vi "pyWebscraper.vi"(8 "error in":errorcluster, 11 "Functions":T1=enum."Check_Ratio") -> (0 "error out":errorcluster, 1 "2D Array":string[][](array[string]), 2 "Standard Output":string, 3 "Output":bool)   [LabVIEW 2025]
uses:
  Control/Function Enum.ctl
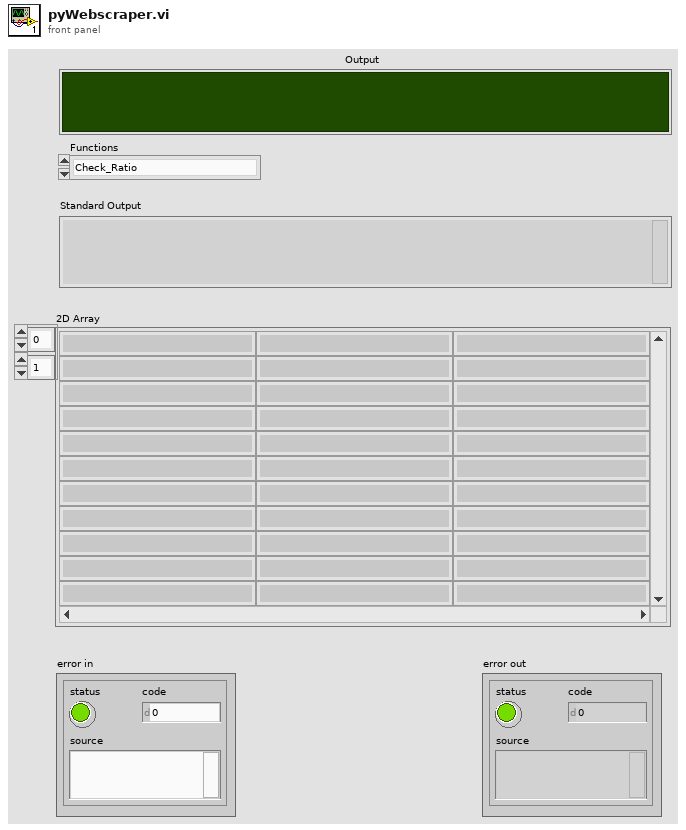
[diagram p1: front panel]
types:
  T1 = typedef "Function Enum.ctl" = enum16{"Check_Config", "Check_Security", "Check_Ratio", "Check_GUI_Loaded", "Read_Overview", "Read_Parameters", "Read_Events", "Read_Alarm", "Read_Settings", "Config_All_Port_Default", "Config_Port1_Speed_10M", "Config_Port1_Speed_100M", "Config_Port2_Speed_10M", "Config_Port2_Speed_100M"}
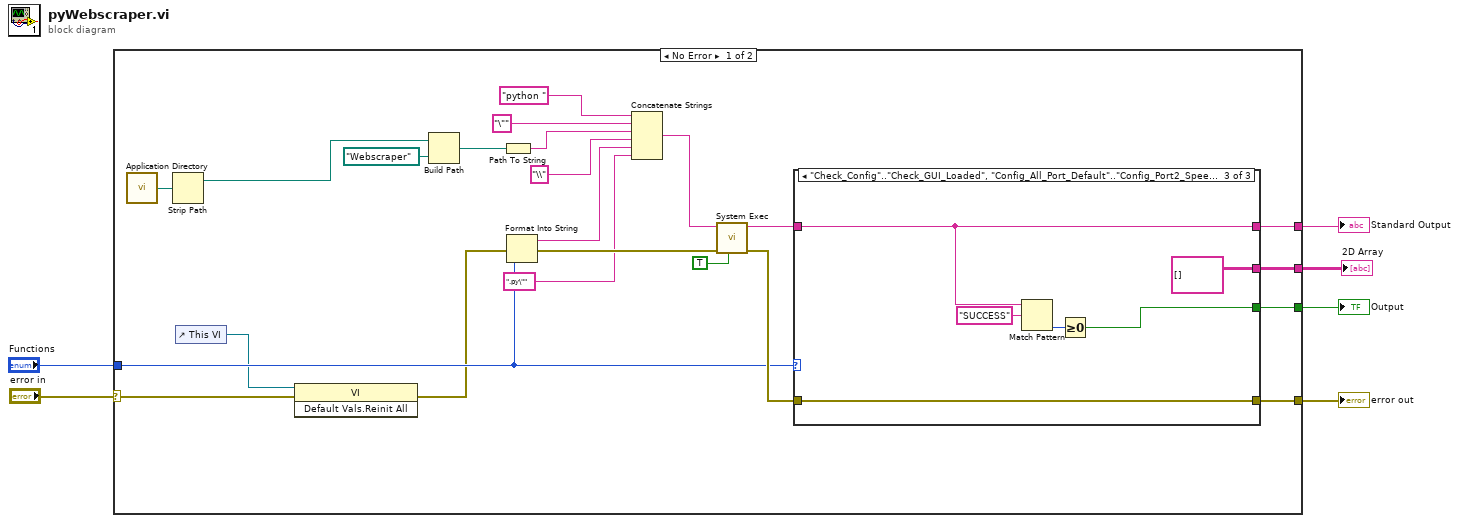
[diagram p0: block diagram]
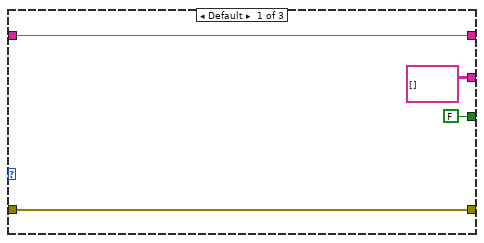
[diagram p2: hidden frame]
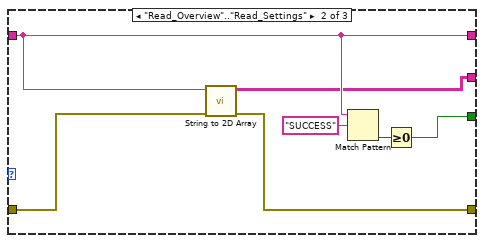
[diagram p3: hidden frame]
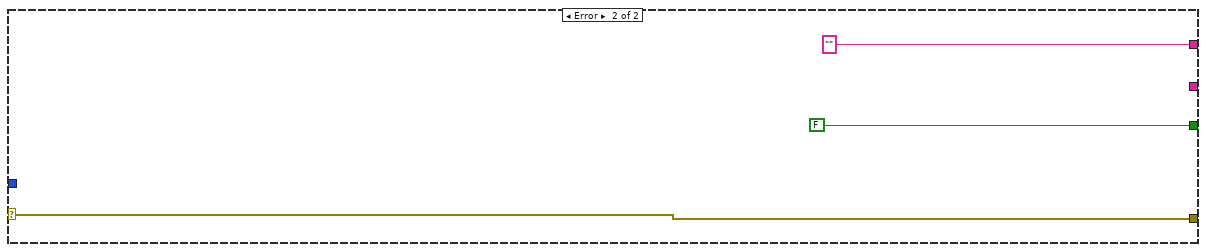
[diagram p4: hidden frame]
diagram:
  n1 = case shown="No Error" "error in" {
    selector: "error in" -> [w8 w49]
    tunnel: [w23 w49] -> w5
    tunnel: "Functions" -> [w22 _]
    tunnel: [w20 "" ("standard output")] -> w4
    tunnel: [w21 FALSE] -> w3
    tunnel: [w19 _] -> w1
    frame No Error {
      n2 = call <vilib>:"Application Directory.vi"() -> ("Application Directory"=w29:path)
      n3 = Strip Path(path=w29) -> (stripped path=w17:path)  [unwired: 1 out]
      n4 = control-ref of="This VI"() -> (w9:refnum<vi>)
      n5 = invoke class="VI" method="Default Vals.Reinit All"(reference=w9, error in=w8) -> (error out=w7:errorcluster)  [unwired: 1 in, 2 out]
      n6 = Build Path(base path=w17, name or relative path=path "Webscraper") -> (appended path=w27:path)
      n7 = Path To String(path=w27) -> (string=w28:string)
      n8 = Format Into String(error in=w7, w22) -> (resulting string=w14:string, error out=w25:errorcluster)  [unwired: 2 in]
      n9 = Concatenate Strings("python " ("string"), "\"" ("string"), w28, "\\" ("string"), w14, ".py\"" ("string")) -> (w10:string)
      n10 = call <vilib>:"System Exec.vi"("run minimized? (F)"=TRUE, "error in (no error)"=w25, "command line"=w10) -> ("error out"=w24:errorcluster, "standard output"=w18:string)  [unwired: 5 in, 2 out]
      n11 = case shown="\"Check_Config\"..\"Check_GUI_Loaded\", \"Config_All_Port_Default\"..\"Config_Port2_Speed_100M\"" w22 {
        tunnel: [FALSE w38 w42] -> w21
        tunnel: w24 -> [w33 w36 w44]
        tunnel: [w33 w37 w44] -> w23
        tunnel: [string[][] [] ("2D Array") w34 string[][] [] ("2D Array")] -> w19
        tunnel: [w32 w35 w41] -> w20
        tunnel: w18 -> [w32 w35 w41]
        frame Default {
        }
        frame "Read_Overview".."Read_Settings" {
          n12 = call "String to 2D Array.vi"("error in (no error)"=w36, "String"=w35) -> ("error out"=w37:errorcluster, "2D Array"=w34:string[][])  [unwired: 8 in]
          n13 = Match Pattern(string=w35, regular expression="SUCCESS") -> (offset past match=w39:i32)  [unwired: 1 in, 3 out]
          n14 = Greater Or Equal To 0?(x=w39) -> (x >= 0?=w38:bool)
        }
        frame "Check_Config".."Check_GUI_Loaded", "Config_All_Port_Default".."Config_Port2_Speed_100M" {
          n15 = Match Pattern(string=w41, regular expression="SUCCESS") -> (offset past match=w45:i32)  [unwired: 1 in, 3 out]
          n16 = Greater Or Equal To 0?(x=w45) -> (x >= 0?=w42:bool)
        }
      }
    }
    frame Error {
    }
  }
  "error out" <- w5
  "Standard Output" <- w4
  "Output" <- w3
  "2D Array" <- w1
